vi "Multi-Instrument Controller.vi"() -> ()   [LabVIEW 2020]
uses:
  Typedefs/Instrument Control.ctl
  Typedefs/Save Params.ctl
  f5f9c0cd-fbfb-4a45-a1ff-eaef7659289b.vi
  <vilib>/Utility/xml.llb/Read From XML File(array).vi
  <vilib>/Utility/file.llb/Write Delimited Spreadsheet (string).vi
  <vilib>/Utility/xml.llb/Write to XML File(string).vi
  <vilib>/Comparison/Less/Less Functor/Less Functor.lvclass
  <instrlib>/Keithley 24XX/Keithley 24XX.lvlib
  <instrlib>/Keithley 648X Series/Keithley 648X Series.lvlib
  <instrlib>/Agilent 34405/Agilent 34405.lvlib
panel:
  out "XY Graph":cluster{dbl[], "Current":dbl[]}[](graph)
  out "rendezvous":T1
  out "Path":path
  in  "Trigger Hardware Address":refnum<visa-resource-name>
  in  "Trigger type":enum16{"Software", "Hardware"}(ring)
  out "start time":dbl
  out "DAQ Timer":string
  in  "Integration Speed":u16(ring)=100 items=["Fast (167µs, 3 digits)"=1, "Med (1.67ms, 4 digits)"=10, "Normal (16.74ms, 5 digits)"=100, "High Accuracy (167ms, 6 digits)"=1000]
  in  "Instrument Config":T2[](array[typedef])
  in  "Running":bool
  in  "Start":bool
  in  "Exit":bool
  in  "Number of Instruments":u64=1 min=1 max=32
  in  "Looping Mode":enum16{"Remote looping", "Local looping"}(ring)
  out "Filename":string
  in  "Stop":bool
  out "Iteration":i32
  in  "Number of Trials\nMax 2500 for remote":i16=300
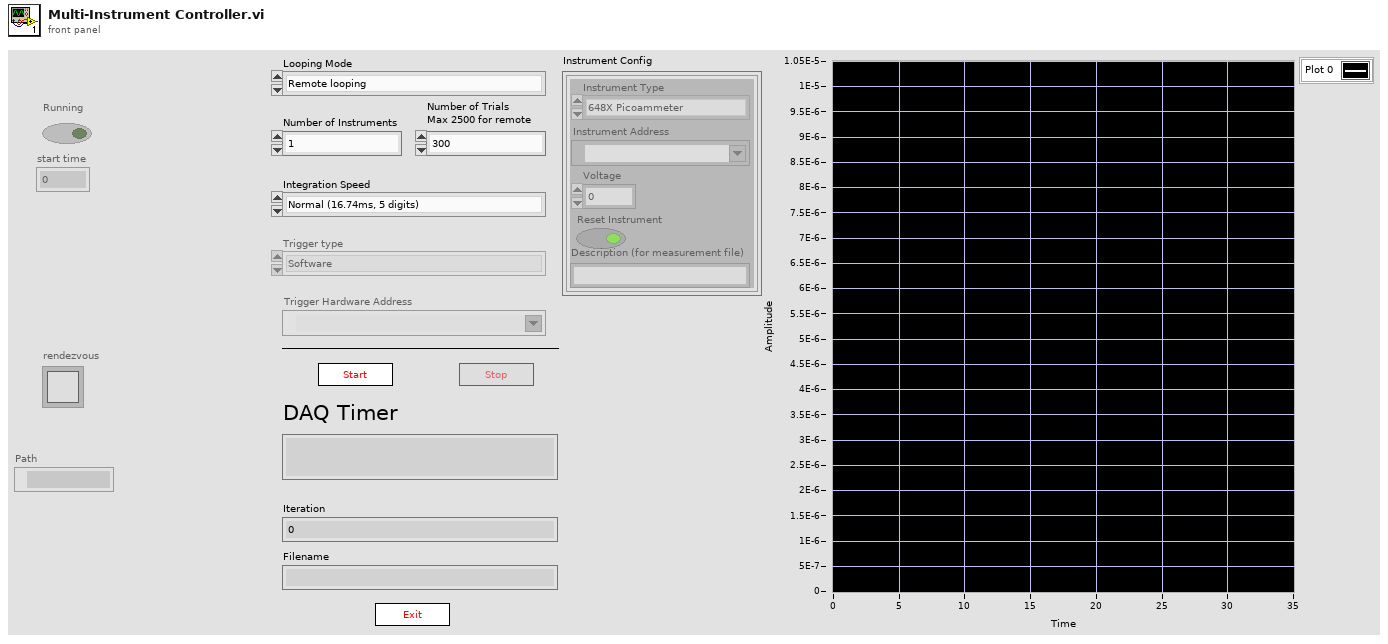
[diagram p1: front panel]
types:
  T1 = typedef "Rendezvous RefNum" = refnum<k1>
  T2 = typedef "Instrument Control.ctl" = cluster{"Instrument Address":refnum<visa-resource-name>, "Voltage":dbl, "Reset Instrument":bool, "Instrument Type":enum16{"648X Picoammeter", "24XX SMU", "237 SMU", "344XX DMM"}, "Description (for measurement file)":string}
  T3 = typedef "Save Params.ctl" = cluster{"Number of Instruments":u64, "Instrument Config":T2[], "Integration Speed":u16, "Measurement Mode":u16, "Number of Trials\nMax 2500 for remote":i16, "Trigger type":enum16{"Software", "Hardware"}, "Trigger Hardware Address":refnum<visa-resource-name>}
  T4 = enum8{"Enabled", "Disabled", "Disabled and Grayed Out"}
  T5 = typedef "LVDateTimeRec.ctl" = cluster{"fractional second":dbl, "second":i32, "minute":i32, "hour":i32, "day of month":i32, "month":i32, "year":i32, "day of week":i32, "day of year":i32, "DST":i32}
  T6 = enum16{"648X Picoammeter", "24XX SMU", "237 SMU", "344XX DMM"}
  T7 = cluster{i32, string[][], cluster{dbl[], "Voltage":sgl[]}, cluster{dbl[], "Current":dbl[]}}
  T8 = cluster{i32, string[][], cluster{dbl[], "Voltage":sgl[]}, cluster{dbl[], "Current":dbl[]}}[]
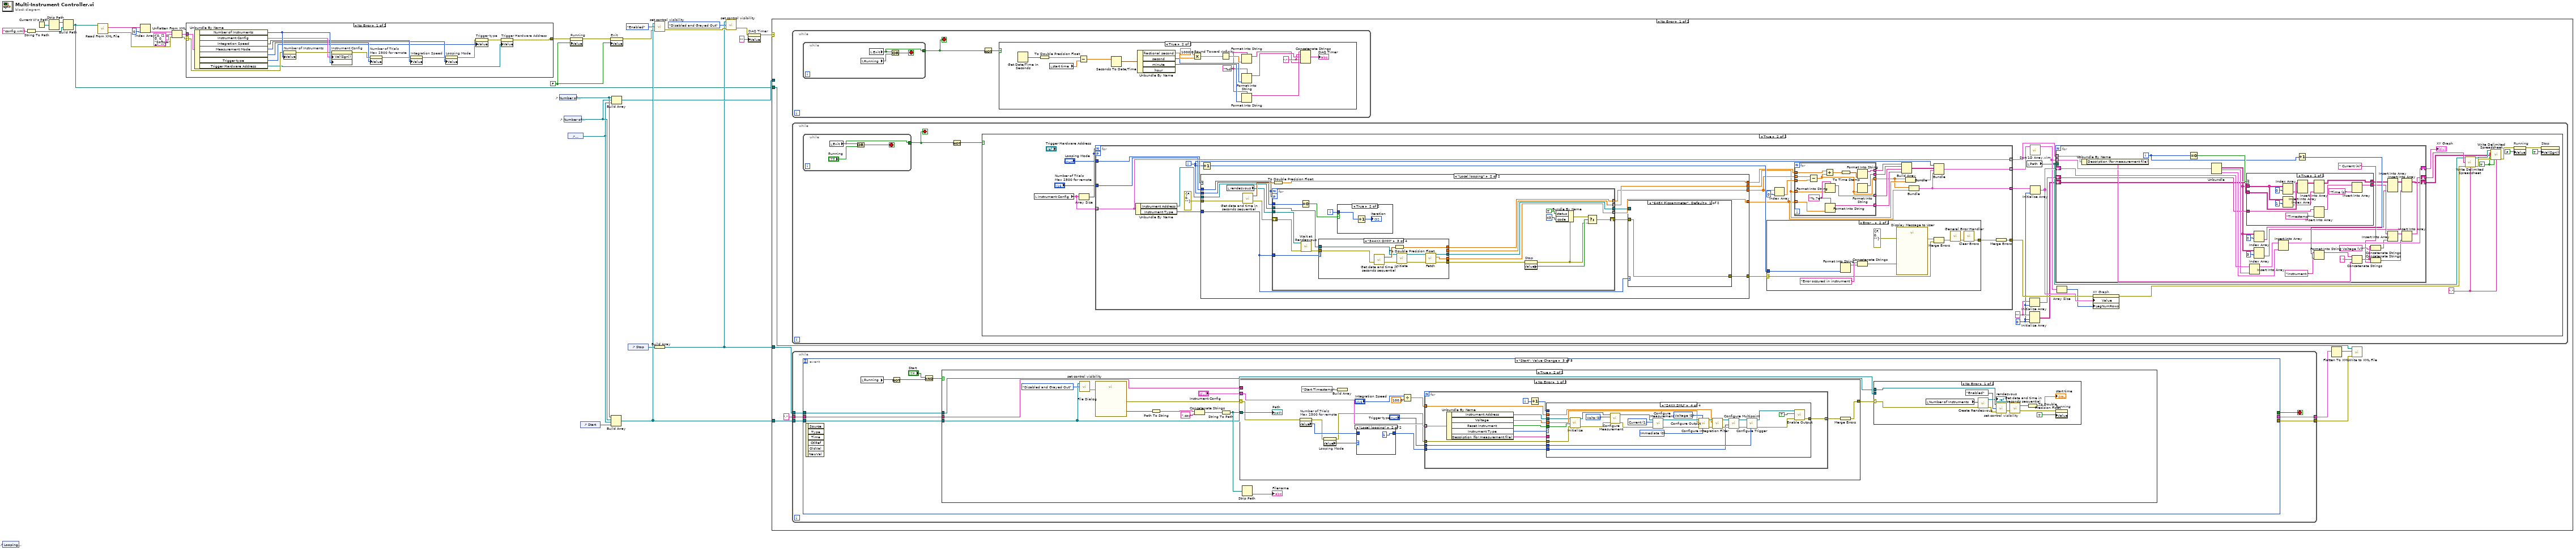
[diagram p0: block diagram]
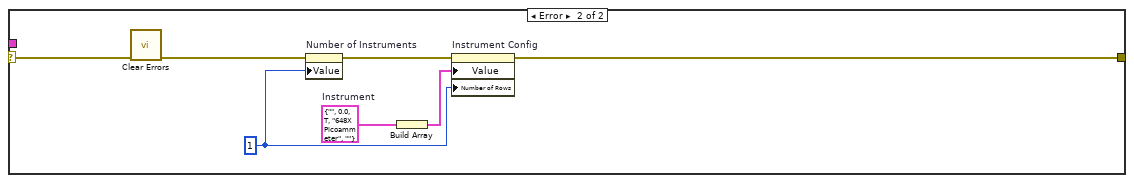
[diagram p2: hidden frame]
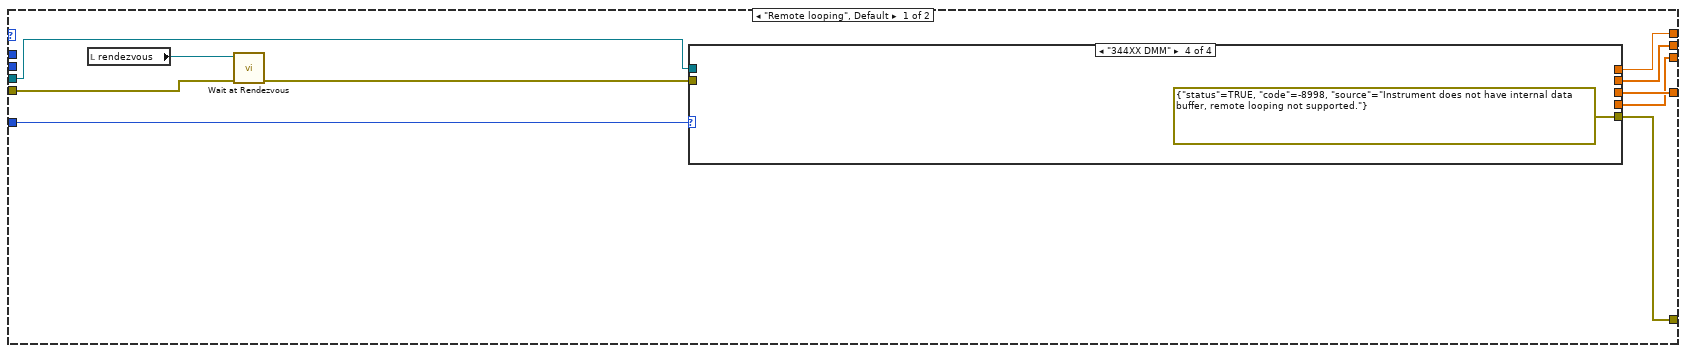
[diagram p6: hidden frame]
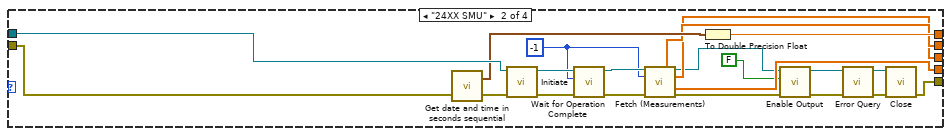
[diagram p8: hidden frame]
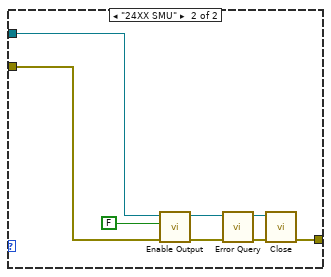
[diagram p10: hidden frame]
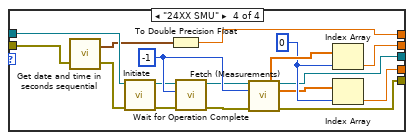
[diagram p13: hidden frame]
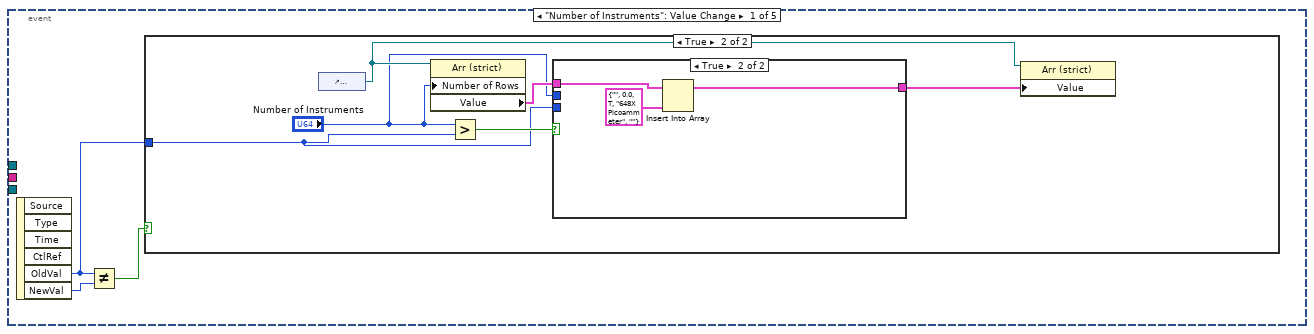
[diagram p16: hidden frame]
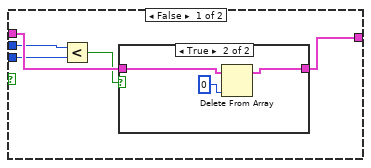
[diagram p18: hidden frame]
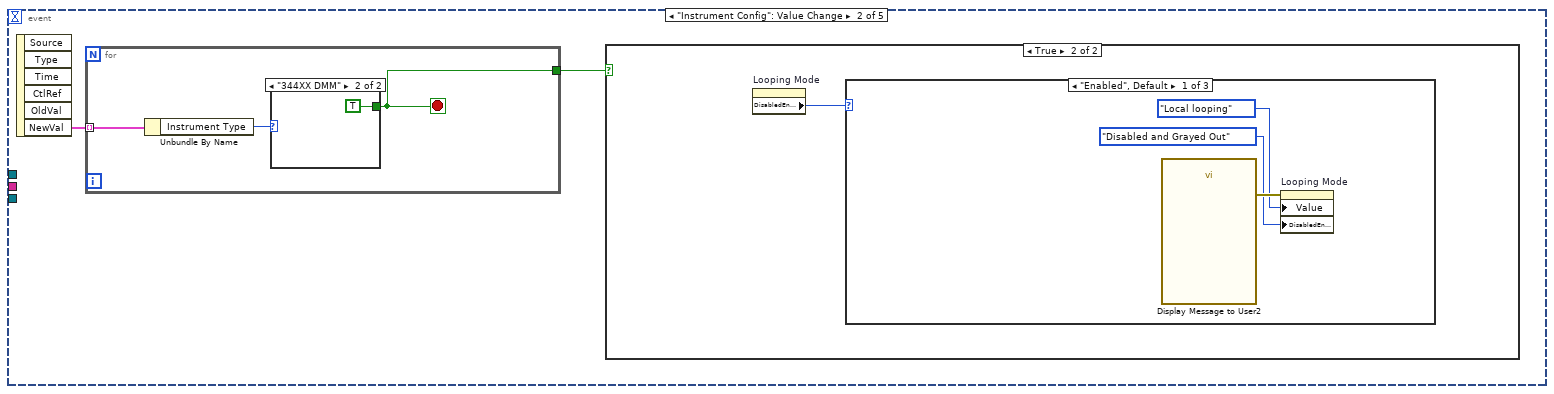
[diagram p20: hidden frame]
diagram:
  w15 = FALSE
  n1 = control-ref of="Looping Mode"() -> ()  [unwired: 1 out]
  n2 = String To Path(string="config.xml") -> (path=w13:path)
  n3 = Current VI's Path() -> (path=w20:path)
  n4 = Strip Path(path=w20) -> (stripped path=w19:path)  [unwired: 1 out]
  n5 = Build Path(base path=w19, name or relative path=w13) -> (appended path=w12:path)
  n6 = call-poly <vilib>:"Read From XML File.vi"("XML File Path"=w12) -> ("error out"=w2:errorcluster, "XML Elements"=w7:string[])  [unwired: 8 in, 1 out]
  n7 = Index Array(array=w7, index=0) -> (element=w4:string)
  n8 = Unflatten From XML(xml string=w4, type=T3 {"Number of Instruments"=0, "Instrument Config"=[], "Integration Speed"=0, "Measurement Mode"=0, "Number of Trials\nMax 2500 for remote"=0, "Trigger type"=enum."Software", "Trigger Hardware Address"=""} ("output cluster"), error in (no error)=w2) -> (value=w3:T3, error out=w1:errorcluster)
  n9 = case shown="No Error" w1 {
    selector: w1 -> [w37 w53]
    tunnel: [w32 w47] -> w9
    tunnel: w3 -> [w31 _]
    frame No Error {
      n10 = Unbundle By Name(w31) -> ("Number of Instruments"=w46:u64, "Instrument Config"=w44:T2[], "Integration Speed"=w40:u16, "Measurement Mode"=w38:u16, "Number of Trials\nMax 2500 for remote"=w42:i16, "Trigger type"=w36:enum16{"Software", "Hardware"}, "Trigger Hardware Address"=w35:refnum<visa-resource-name>)
      n11 = property on="Number of Instruments" class="DigNum (strict)"(error in=w37, "Value"=w46) -> (error out=w45:errorcluster)  [unwired: 1 in, 1 out]
      n12 = property on="Instrument Config" class="Arr (strict)"(error in=w45, "Val(Sgnl)"=w44, "Number of Rows"=w46) -> (error out=w43:errorcluster)  [unwired: 1 in, 1 out]
      n13 = property on="Number of Trials\nMax 2500 for remote" class="DigNum (strict)"(error in=w43, "Value"=w42) -> (error out=w41:errorcluster)  [unwired: 1 in, 1 out]
      n14 = property on="Integration Speed" class="Ring (strict)"(error in=w41, "Value"=w40) -> (error out=w39:errorcluster)  [unwired: 1 in, 1 out]
      n15 = property on="Looping Mode" class="Enum (strict)"(error in=w39, "Value"=w38) -> (error out=w34:errorcluster)  [unwired: 1 in, 1 out]
      n16 = property on="Trigger type" class="Enum (strict)"(error in=w34, "Value"=w36) -> (error out=w33:errorcluster)  [unwired: 1 in, 1 out]
      n17 = property on="Trigger Hardware Address" class="VISAName"(error in=w33, "Value"=w35) -> (error out=w32:errorcluster)  [unwired: 1 in, 1 out]
    }
    frame Error {
      w50 = T2 {"Instrument Address"="", "Voltage"=0.0, "Reset Instrument"=TRUE, "Instrument Type"=enum."648X Picoammeter", "Description (for measurement file)"=""}  # Instrument
      w51 = 1
      n18 = call <vilib>:"Clear Errors.vi"("error in (no error)"=w53) -> ("error out"=w52:errorcluster)  [unwired: 5 in, 1 out]
      n19 = property on="Number of Instruments" class="DigNum (strict)"(error in=w52, "Value"=w51) -> (error out=w48:errorcluster)  [unwired: 1 in, 1 out]
      n20 = Build Array(w50) -> (w49:T2[])
      n21 = property on="Instrument Config" class="Arr (strict)"(error in=w48, "Value"=w49, "Number of Rows"=w51) -> (error out=w47:errorcluster)  [unwired: 1 in, 1 out]
    }
  }
  n22 = control-ref of="Number of Instruments"() -> (w23:refnum<vi>)
  n23 = control-ref of="Number of Trials\nMax 2500 for remote"() -> (w22:refnum<vi>)
  n24 = control-ref of="Instrument Config"() -> (w21:refnum<vi>)
  n25 = property on="Running" class="Bool (strict)"(error in=w9, "Value"=w15) -> (error out=w14:errorcluster)  [unwired: 1 in, 1 out]
  n26 = control-ref of="Start"() -> (w29:refnum<vi>)
  n27 = property on="Exit" class="Bool (strict)"(error in=w14, "Value"=w15) -> (error out=w24:errorcluster)  [unwired: 1 in, 1 out]
  n28 = Build Array(w23, w22, w21, w29) -> (w25:refnum<vi>[])
  n29 = Build Array(w23, w22, w21) -> (w17:refnum<vi>[])
  n30 = control-ref of="Stop"() -> (w28:refnum<vi>)
  n31 = call "set control visibility.vi"("error in"=w24, "Disabled"=T4."Enabled", "Controls Reference Array"=w25) -> ("error out"=w27:errorcluster)  [unwired: 1 in]
  n32 = Build Array(w28) -> (w16:refnum<vi>[])
  n33 = call "set control visibility.vi"("error in"=w27, "Disabled"=T4."Disabled and Grayed Out", "Controls Reference Array"=w16) -> ("error out"=w8:errorcluster)  [unwired: 1 in]
  n34 = property on="DAQ Timer" class="Str"(error in=w8, "Value"="") -> (error out=w10:errorcluster)  [unwired: 1 in, 1 out]
  n35 = case shown="No Error" w10 {
    selector: w10 -> [_ w514]
    tunnel: w25 -> [w59 _]
    tunnel: w12 -> [w55 _]
    tunnel: w17 -> [_ _]
    tunnel: w16 -> [w54 _]
    frame No Error {
      n36 = while {
        stop <- w61 stop-if-true
        n37 = while {
          tunnel: [w80] -> w61
          stop <- w81 stop-if-true
          n38 = local read "Running"() -> (w82:bool)
          n39 = local read "Exit"() -> (w80:bool)
          n40 = Or(x=w80, y=w82) -> (x .or. y?=w81:bool)
        }
        n41 = Not(x=w61) -> (.not. x?=w62:bool)
        n42 = case shown="True" w62 {
          frame False {
          }
          frame True {
            w64 = "%d" ("format string")
            w69 = ":"
            n43 = Get Date/Time In Seconds() -> (seconds since 1Jan1904=w66:timestamp)
            n44 = To Double Precision Float(number=w66) -> (double precision float=w65:dbl)
            n45 = local read "start time"() -> (w63:dbl)
            n46 = Subtract(x=w65, y=w63) -> (x-y=w79:dbl)
            n47 = Seconds To Date/Time(time stamp (now)=w79) -> (date time rec=w78:T5)  [unwired: 1 in]
            n48 = Unbundle By Name(w78) -> ("fractional second"=w77:dbl, "second"=w73:i32, "minute"=w72:i32)  [unwired: 1 out]
            n49 = Multiply(x=1000.0, y=w77) -> (x*y=w75:dbl)
            n50 = Round Toward -Infinity(1:w75) -> (0:w74:dbl)
            n51 = Format Into String(format string=w64, w74) -> (resulting string=w68:string)  [unwired: 2 in, 1 out]
            n52 = Format Into String(format string=w64, w73) -> (resulting string=w70:string)  [unwired: 2 in, 1 out]
            n53 = Format Into String(format string=w64, w72) -> (resulting string=w71:string)  [unwired: 2 in, 1 out]
            n54 = Concatenate Strings(w71, w69, w70, w69, w68) -> (→"DAQ Timer":string)
          }
        }
      }
      n55 = while {
        stop <- w83 stop-if-true
        n56 = while {
          tunnel: [w316] -> w83
          stop <- w317 stop-if-true
          n57 = local read "Exit"() -> (w316:bool)
          n58 = Or(x=w316, y="Running") -> (x .or. y?=w317:bool)
        }
        n59 = Not(x=w83) -> (.not. x?=w84:bool)
        n60 = case shown="True" w84 {
          frame False {
          }
          frame True {
            w90 = ","
            w92 = TRUE ("transpose? (no:F)")
            w87 = ""
            w86 = 0 ("dimension size")
            n61 = local read "Instrument Config"() -> (w111:T2[])
            n62 = Array Size(array=w111) -> (size(s)=w112:i32)
            n63 = for {
              N: w112 -> [_]
              workers-P: w112 -> [_]
              tunnel: w111 -> [w172] mode=indexing
              tunnel: [w175] -> w100
              tunnel: [w173] -> w110 mode=indexing
              tunnel: [w172] -> w109 mode=indexing
              tunnel: "Looping Mode" -> [w171]
              tunnel: "Number of Trials\nMax 2500 for remote" -> [w170]
              tunnel: [w164] -> w103
              i -> [w169]
              n64 = Unbundle By Name(w172) -> ("Instrument Address"=w163:refnum<visa-resource-name>, "Instrument Type"=w161:T6)
              n65 = case shown="\"Local looping\"" w171 {
                tunnel: w163 -> [w191 w227]
                tunnel: [w190 w231] -> w184
                tunnel: [w189 w230] -> w168
                tunnel: [w188 w229] -> w166
                tunnel: [w187 w228] -> w182
                tunnel: errorcluster {"status"=FALSE, "code"=0, "source"=""} ("error constant") -> [w195 w226]
                tunnel: [w186 w221] -> w160
                tunnel: w170 -> [_ w219]
                tunnel: w169 -> [_ w223]
                tunnel: w161 -> [w193 w220]
                frame "Remote looping", Default {
                  n66 = local read "rendezvous"() -> (w194:T1)
                  n67 = call <vilib>:"Wait at Rendezvous.vi"("error in (no error)"=w195, "rendezvous"=w194) -> ("error out"=w192:errorcluster)  [unwired: 3 in, 2 out]
                  n68 = case shown="\"344XX DMM\"" w193 {
                    tunnel: w192 -> [_ w198 _ _]
                    tunnel: w191 -> [_ w216 _ _]
                    tunnel: [_ w214 _ _] -> w190
                    tunnel: [_ w210 _ _] -> w189
                    tunnel: [_ w209 _ _] -> w188
                    tunnel: [_ w208 _ _] -> w187
                    tunnel: [_ w199 _ errorcluster {"status"=TRUE, "code"=-8998, "source"="Instrument does not have internal data buffer, remote looping not supported."} ("error constant")] -> w186
                    frame "648X Picoammeter", Default {
                    }
                    frame "24XX SMU" {
                      w207 = -1
                      n69 = call "Get date and time in seconds sequential.vi"("error in (no error)"=w198) -> ("error out"=w197:errorcluster, "current time"=w215:timestamp)  [unwired: 1 in]
                      n70 = call <instrlib>:"Initiate.vi"("error in (no error)"=w197, "VISA resource name"=w216) -> ("error out"=w196:errorcluster, "VISA resource name out"=w213:refnum<visa-resource-name>)  [unwired: 8 in]
                      n71 = call <instrlib>:"Wait for Operation Complete.vi"("error in (no error)"=w196, "Timeout (10000 ms)"=w207, "VISA resource name"=w213) -> ("error out"=w211:errorcluster, "VISA resource name out"=w212:refnum<visa-resource-name>)  [unwired: 7 in]
                      n72 = call <instrlib>:"Fetch (Measurements).vi"("VISA resource name"=w212, "Timeout (10000 ms)"=w207, "error in (no error)"=w211) -> ("Voltage"=w210:sgl[], "VISA resource name out"=w206:refnum<visa-resource-name>, "Current"=w209:sgl[], "Timestamp"=w208:sgl[], "error out"=w205:errorcluster)  [unwired: 6 in, 2 out]
                      n73 = To Double Precision Float(number=w215) -> (double precision float=w214:dbl)
                      n74 = call <instrlib>:"Enable Output.vi"("error in (no error)"=w205, "Enable Output (T: Enable)"=FALSE, "VISA resource name"=w206) -> ("error out"=w202:errorcluster, "VISA resource name out"=w203:refnum<visa-resource-name>)  [unwired: 7 in]
                      n75 = call <instrlib>:"Error Query.vi"("error in (no error)"=w202, "VISA resource name"=w203) -> ("error out"=w200:errorcluster, "VISA resource name out"=w201:refnum<visa-resource-name>)  [unwired: 6 in, 2 out]
                      n76 = call <instrlib>:"Close.vi"("error in (no error)"=w200, "VISA resource name"=w201) -> ("error out"=w199:errorcluster)  [unwired: 9 in]
                    }
                    frame "237 SMU" {
                    }
                    frame "344XX DMM" {
                    }
                  }
                }
                frame "Local looping" {
                  n77 = local read "rendezvous"() -> (w224:T1)
                  n78 = call "Get date and time in seconds sequential.vi"("error in (no error)"=w226) -> ("error out"=w225:errorcluster, "current time"=w232:timestamp)  [unwired: 1 in]
                  n79 = for {
                    N: w219 -> [_]
                    tunnel: [w260] -> w230 mode=indexing
                    tunnel: [w259] -> w229 mode=indexing
                    tunnel: [w252] -> w228 mode=indexing
                    tunnel: w227 -> [w258]
                    tunnel: [w257] -> w222
                    tunnel: w224 -> [w251]
                    tunnel: w223 -> [w255]
                    tunnel: w220 -> [w253]
                    workers-P: w219 -> [_]
                    shift-right: [w244] -> w218
                    shift-left: w225 -> [w250]
                    i -> [w256]
                    n80 = Equal To 0?(x=w255) -> (x = 0?=w254:bool)
                    n81 = call <vilib>:"Wait at Rendezvous.vi"("error in (no error)"=w250, "rendezvous"=w251) -> ("error out"=w249:errorcluster)  [unwired: 3 in, 2 out]
                    n82 = case shown="\"344XX DMM\"" w253 {
                      tunnel: w249 -> [w261 w262 w265 w275]
                      tunnel: [_ _ _ w286] -> w260
                      tunnel: [_ _ w267 w283] -> w259
                      tunnel: w258 -> [_ _ w269 w282]
                      tunnel: [_ _ w268 w279] -> w257
                      tunnel: [w261 w262 w266 w278] -> w248
                      tunnel: [_ _ w271 w276] -> w252
                      frame "648X Picoammeter", Default {
                      }
                      frame "237 SMU" {
                      }
                      frame "344XX DMM" {
                        n83 = call "Get date and time in seconds sequential.vi"("error in (no error)"=w265) -> ("error out"=w264:errorcluster, "current time"=w272:timestamp)  [unwired: 1 in]
                        n84 = To Double Precision Float(number=w272) -> (double precision float=w271:dbl)
                        n85 = call <instrlib>:"Initiate.vi"("error in (no error)"=w264, "VISA resource name"=w269) -> ("error out"=w263:errorcluster, "VISA resource name out"=w270:refnum<visa-resource-name>)  [unwired: 8 out]
                        n86 = call <instrlib>:"Fetch.vi"("error in (no error)"=w263, "VISA resource name"=w270) -> ("error out"=w266:errorcluster, "Measurement"=w267:dbl, "VISA resource name out"=w268:refnum<visa-resource-name>)  [unwired: 7 out]
                      }
                      frame "24XX SMU" {
                        w285 = 0
                        w288 = -1
                        n87 = call "Get date and time in seconds sequential.vi"("error in (no error)"=w275) -> ("error out"=w274:errorcluster, "current time"=w277:timestamp)  [unwired: 1 in]
                        n88 = call <instrlib>:"Initiate.vi"("error in (no error)"=w274, "VISA resource name"=w282) -> ("error out"=w273:errorcluster, "VISA resource name out"=w281:refnum<visa-resource-name>)  [unwired: 8 in]
                        n89 = To Double Precision Float(number=w277) -> (double precision float=w276:dbl)
                        n90 = call <instrlib>:"Wait for Operation Complete.vi"("error in (no error)"=w273, "Timeout (10000 ms)"=w288, "VISA resource name"=w281) -> ("error out"=w289:errorcluster, "VISA resource name out"=w280:refnum<visa-resource-name>)  [unwired: 7 in]
                        n91 = call <instrlib>:"Fetch (Measurements).vi"("VISA resource name"=w280, "Timeout (10000 ms)"=w288, "error in (no error)"=w289) -> ("Voltage"=w287:sgl[], "VISA resource name out"=w279:refnum<visa-resource-name>, "Current"=w284:sgl[], "error out"=w278:errorcluster)  [unwired: 6 in, 3 out]
                        n92 = Index Array(array=w287, index=w285) -> (element=w286:sgl)
                        n93 = Index Array(array=w284, index=w285) -> (element=w283:sgl)
                      }
                    }
                    n94 = case shown="True" w254 {
                      tunnel: w256 -> [_ w291]
                      frame False {
                      }
                      frame True {
                        n95 = Increment(x=w291) -> (x+1=→"Iteration":i32)
                      }
                    }
                    n96 = property on="Stop" class="Bool (strict)"(error in=w248) -> (error out=w243:errorcluster, "Value"=w247:bool)  [unwired: 1 in, 1 out]
                    n97 = Bundle By Name(cluster=w243, "status"=TRUE, "code"=43) -> (w242:errorcluster)
                    n98 = Select(t=w242, s=w247, f=w243) -> (s? t:f=w244:errorcluster)
                  }
                  n99 = To Double Precision Float(number=w232) -> (double precision float=w231:dbl)
                  n100 = case shown="\"648X Picoammeter\", Default" w220 {
                    tunnel: w222 -> [_ w237]
                    tunnel: [w233 w236] -> w221
                    tunnel: w218 -> [w233 w234]
                    frame "648X Picoammeter", Default {
                    }
                    frame "24XX SMU" {
                      n101 = call <instrlib>:"Enable Output.vi"("error in (no error)"=w234, "Enable Output (T: Enable)"=FALSE, "VISA resource name"=w237) -> ("error out"=w240:errorcluster, "VISA resource name out"=w241:refnum<visa-resource-name>)  [unwired: 7 in]
                      n102 = call <instrlib>:"Error Query.vi"("error in (no error)"=w240, "VISA resource name"=w241) -> ("error out"=w238:errorcluster, "VISA resource name out"=w239:refnum<visa-resource-name>)  [unwired: 6 in, 2 out]
                      n103 = call <instrlib>:"Close.vi"("error in (no error)"=w238, "VISA resource name"=w239) -> ("error out"=w236:errorcluster)  [unwired: 9 in]
                    }
                  }
                }
              }
              n104 = Increment(x=w169) -> (x+1=w185:i32)
              n105 = case shown="Error .." w160 {
                selector: w160 -> [w305 w309]
                tunnel: [w305 w306] -> w180
                tunnel: w185 -> [_ w314]
                frame No Error {
                }
                frame Error {
                  n106 = Format Into String(w314) -> (resulting string=w313:string)  [unwired: 3 in, 1 out]
                  n107 = Concatenate Strings("Error occured in instrument " ("Message"), w313) -> (w312:string)
                  n108 = call "Display Message to User"("error in (no error)"=errorcluster {"status"=FALSE, "code"=0, "source"=""} ("error constant"), "Message"=w312) -> ("error out"=w310:errorcluster)  [unwired: 8 in, 1 out]
                  n109 = Merge Errors(w310, w309) -> (w308:errorcluster)
                  n110 = call <vilib>:"General Error Handler.vi"("error in (no error)"=w308) -> ("error out"=w307:errorcluster)  [unwired: 10 in, 4 out]
                  n111 = call <vilib>:"Clear Errors.vi"("error in (no error)"=w307) -> ("error out"=w306:errorcluster)  [unwired: 5 in, 1 out]
                }
              }
              n112 = Index Array(array=w182, index=0) -> (element=w181:dbl)
              n113 = for {
                tunnel: [w304] -> w176 mode=indexing
                tunnel: [w303] -> w177 mode=indexing
                tunnel: w182 -> [w302] mode=indexing
                tunnel: w168 -> [w292] mode=indexing
                tunnel: w181 -> [w301]
                tunnel: w166 -> [w294] mode=indexing
                tunnel: w184 -> [w299]
                tunnel: [w296] -> w179 mode=indexing
                tunnel: [w295] -> w178 mode=indexing
                tunnel: [w293] -> w167 mode=indexing
                w300 = "%.7e"
                n114 = Subtract(x=w302, y=w301) -> (x-y=w293:dbl)
                n115 = Add(x=w299, y=w293) -> (x+y=w298:dbl)
                n116 = Format Into String(format string=w300, w292) -> (resulting string=w303:string)  [unwired: 2 in, 1 out]
                n117 = Format Into String(format string=w300, w294) -> (resulting string=w304:string)  [unwired: 2 in, 1 out]
                n118 = To Time Stamp(1:w298) -> (0:w297:timestamp)
                n119 = Format Into String(w297) -> (resulting string=w296:string)  [unwired: 3 in, 1 out]
                n120 = Format Into String(w293) -> (resulting string=w295:string)  [unwired: 3 in, 1 out]
              }
              n121 = Build Array(w179, w178, w177, w176) -> (w174:string[][])
              n122 = Bundle(w167, "Voltage"=w168) -> (w165:cluster{dbl[], "Voltage":sgl[]})  [unwired: 1 in]
              n123 = Bundle(w167, "Current"=w166) -> (w164:cluster{dbl[], "Current":dbl[]})  [unwired: 1 in]
              n124 = Bundle(w169, w174, w165, w164) -> (w173:T7)  [unwired: 1 in]
              n125 = Merge Errors(w180) -> (w175:errorcluster)
            }
            n126 = local read "Path"() -> (w94:path)
            n127 = Initialize Array(w87, w86) -> (w97:string[])
            n128 = Initialize Array(w87, w86, w86) -> (w88:string[][])
            n129 = call "Sort 1D Array.vim"("unsorted array"=w110) -> ("sorted array"=w99:T8)  [unwired: 10 in]
            n130 = Initialize Array(w103, w86) -> (w101:cluster{dbl[], "Current":dbl[]}[])
            n131 = for {
              tunnel: w99 -> [w144] mode=indexing
              tunnel: w109 -> [w143] mode=indexing
              tunnel: w94 -> [_]
              shift-right: [w133] -> w102
              shift-left: w101 -> [w137]
              shift-right: [w122] -> w95
              shift-left: w97 -> [w127]
              shift-right: [w113] -> w85
              shift-left: w88 -> [w121]
              i -> [w128]
              n132 = Unbundle By Name(w143) -> ("Description (for measurement file)"=w131:string)
              n133 = Equal To 0?(x=w128) -> (x = 0?=w129:bool)
              n134 = Unbundle(w144) -> (w117:string[][], w136:cluster{dbl[], "Voltage":sgl[]}, w134:cluster{dbl[], "Current":dbl[]})  [unwired: 1 out]
              n135 = case shown="True" w129 {
                tunnel: w127 -> [w146 w159]
                tunnel: [w146 w155] -> w126
                tunnel: w121 -> [w145 w154]
                tunnel: [w145 w152] -> w118
                tunnel: w117 -> [_ w147]
                frame False {
                }
                frame True {
                  n136 = Index Array(array=w147, index (row)=0) -> (element=w150:string[])  [unwired: 1 in]
                  n137 = Index Array(array=w147, index (row)=1) -> (element=w148:string[])  [unwired: 1 in]
                  n138 = Insert Into Array(array=w154, new element=w150) -> (w153:string[][])  [unwired: 2 in]
                  n139 = Insert Into Array(array=w153, new element=w148) -> (w152:string[][])  [unwired: 2 in]
                  n140 = Insert Into Array(array=w159, new element="Timestamp") -> (w157:string[])  [unwired: 1 in]
                  n141 = Insert Into Array(array=w157, new element="Time (s)") -> (w155:string[])  [unwired: 1 in]
                }
              }
              n142 = Insert Into Array(array=w137, new element=w136) -> (w135:cluster{dbl[], "Current":dbl[]}[])  [unwired: 1 in]
              n143 = Index Array(array=w117, index (row)=2) -> (element=w116:string[])  [unwired: 1 in]
              n144 = Index Array(array=w117, index (row)=3) -> (element=w114:string[])  [unwired: 1 in]
              n145 = Insert Into Array(array=w135, new element=w134) -> (w133:cluster{dbl[], "Current":dbl[]}[])  [unwired: 1 in]
              n146 = Increment(x=w128) -> (x+1=w142:i32)
              n147 = Format Into String(initial string="Instrument ", w142) -> (resulting string=w140:string)  [unwired: 2 in, 1 out]
              n148 = Concatenate Strings(w140, " ", w131) -> (w138:string)
              n149 = Concatenate Strings(w138, " Voltage (V)") -> (w125:string)
              n150 = Concatenate Strings(w138, " Current (A)") -> (w124:string)
              n151 = Insert Into Array(array=w118, new element=w116) -> (w115:string[][])  [unwired: 2 in]
              n152 = Insert Into Array(array=w126, new element=w125) -> (w123:string[])  [unwired: 1 in]
              n153 = Insert Into Array(array=w115, new element=w114) -> (w113:string[][])  [unwired: 2 in]
              n154 = Insert Into Array(array=w123, new element=w124) -> (w122:string[])  [unwired: 1 in]
            }
            "XY Graph" <- w102
            n155 = Array Size(array=w99) -> (size(s)=w98:i32)
            n156 = property on="XY Graph" class="XYGraph (strict)"(error in=w100, "Value"=w101, "LegNumRows"=w98) -> (error out=w96:errorcluster)  [unwired: 1 in, 1 out]
            n157 = call-poly <vilib>:"Write Delimited Spreadsheet.vi"("file path (dialog if empty)"=w94, "1D data"=w95, "error in (no error)"=w96, "delimiter (\\t)"=w90) -> ("new file path (Not A Path if cancelled)"=w91:path, "error out"=w93:errorcluster)  [unwired: 10 in]
            n158 = call-poly <vilib>:"Write Delimited Spreadsheet.vi"("file path (dialog if empty)"=w91, "2D data"=w85, "append to file? (new file:F)"=w92, "error in (no error)"=w93, "transpose? (no:F)"=w92, "delimiter (\\t)"=w90) -> ("error out"=w89:errorcluster)  [unwired: 8 in, 1 out]
            n159 = property on="Running" class="Bool (strict)"(error in=w89, "Value"=FALSE) -> (error out=w106:errorcluster)  [unwired: 1 in, 1 out]
            n160 = property on="Stop" class="Bool (strict)"(error in=w106, "Val(Sgnl)"=TRUE) -> ()  [unwired: 1 in, 2 out]
          }
        }
      }
      n161 = while {
        tunnel: "," -> [w323]
        tunnel: w59 -> [w322]
        tunnel: [w321] -> w58
        tunnel: [w320] -> w56
        tunnel: w54 -> [w319]
        stop <- w324 stop-if-true
        n162 = event shown="[2] \"Start\": Value Change" {
          selector: _ -> [_ _ _ _ _]
          dyn-events: _ -> [_ _ _ _ _]
          timeout: _ -> [_ _ _ _ _]
          tunnel: [_ _ _ _ "Exit"] -> w324
          tunnel: w323 -> [_ _ w360 _ _]
          tunnel: w322 -> [_ _ w359 w471 _]
          tunnel: [_ _ _ _ w507] -> w321
          tunnel: [_ _ _ _ errorcluster {"status"=FALSE, "code"=0, "source"=""} ("error constant")] -> w320
          tunnel: w319 -> [_ _ w358 w467 _]
          event "Number of Instruments": Value Change {
            n163 = event-data() -> ("OldVal"=w325:u64, "NewVal"=w327:u64)  [unwired: 1 in, 4 out]
            n164 = Not Equal?(x=w325, y=w327) -> (x != y?=w326:bool)
            n165 = case shown="True" w326 {
              tunnel: w325 -> [_ w328]
              frame False {
              }
              frame True {
                n166 = control-ref of="Instrument Config"() -> (w330:refnum<vi>)
                n167 = property on="Property Node" class="Arr (strict)"(reference=w330, "Number of Rows"="Number of Instruments") -> ("Value"=w332:T2[])  [unwired: 1 in, 2 out]
                n168 = Greater?(x="Number of Instruments", y=w328) -> (0:w333:bool)
                n169 = case shown="True" w333 {
                  tunnel: w332 -> [w338 w345]
                  tunnel: [w337 w344] -> w331
                  tunnel: "Number of Instruments" -> [w336 _]
                  tunnel: w328 -> [w335 _]
                  frame False {
                    n170 = Less?(x=w336, y=w335) -> (x < y?=w334:bool)
                    n171 = case shown="True" w334 {
                      tunnel: w338 -> [w339 w342]
                      tunnel: [w339 w341] -> w337
                      frame False {
                      }
                      frame True {
                        n172 = Delete From Array(array=w342, index=0) -> (array with subset deleted=w341:T2[])  [unwired: 1 in, 1 out]
                      }
                    }
                  }
                  frame True {
                    n173 = Insert Into Array(array=w345, new element=T2 {"Instrument Address"="", "Voltage"=0.0, "Reset Instrument"=TRUE, "Instrument Type"=enum."648X Picoammeter", "Description (for measurement file)"=""}) -> (w344:T2[])  [unwired: 1 in]
                  }
                }
                n174 = property on="Property Node" class="Arr (strict)"(reference=w330, "Value"=w331) -> ()  [unwired: 1 in, 2 out]
              }
            }
          }
          event "Instrument Config": Value Change {
            n175 = event-data() -> ("NewVal"=w347:T2[])  [unwired: 1 in, 5 out]
            n176 = for {
              tunnel: w347 -> [w355] mode=indexing
              tunnel: [w353] -> w346
              stop <- w353 stop-if-true
              n177 = Unbundle By Name(w355) -> ("Instrument Type"=w354:T6)
              n178 = case shown="\"344XX DMM\"" w354 {
                tunnel: [FALSE TRUE] -> w353
                frame "648X Picoammeter", Default {
                }
                frame "344XX DMM" {
                }
              }
            }
            n179 = case shown="True" w346 {
              frame False {
                n180 = property on="Looping Mode" class="Enum (strict)"("DisabledEnum"=T4."Enabled" ("Disabled")) -> ()  [unwired: 2 in, 2 out]
              }
              frame True {
                n181 = property on="Looping Mode" class="Enum (strict)"() -> ("DisabledEnum"=w349:T4)  [unwired: 2 in, 2 out]
                n182 = case shown="\"Enabled\", Default" w349 {
                  frame "Enabled", Default {
                    n183 = call "Display Message to User2"() -> ("error out"=w352:errorcluster)  [unwired: 10 in, 1 out]
                    n184 = property on="Looping Mode" class="Enum (strict)"(error in=w352, "Value"=enum16{"Remote looping", "Local looping"}."Local looping" ("Looping Mode"), "DisabledEnum"=T4."Disabled and Grayed Out" ("Disabled")) -> ()  [unwired: 1 in, 2 out]
                  }
                  frame "Disabled" {
                  }
                  frame "Disabled and Grayed Out" {
                  }
                }
              }
            }
          }
          event "Start": Value Change {
            n185 = event-data() -> ()  [unwired: 1 in, 6 out]
            n186 = local read "Running"() -> (w364:bool)
            n187 = Not(x=w364) -> (.not. x?=w363:bool)
            n188 = And(x="Start", y=w363) -> (x .and. y?=w361:bool)
            n189 = case shown="True" w361 {
              tunnel: w360 -> [_ w372]
              tunnel: w359 -> [_ w367]
              tunnel: w358 -> [_ w366]
              frame False {
              }
              frame True {
                n190 = call "set control visibility.vi"("Disabled"=T4."Disabled and Grayed Out", "Controls Reference Array"=w367) -> ("error out"=w369:errorcluster)  [unwired: 2 in]
                n191 = call "File Dialog"("error in"=w369) -> ("selected path"=w375:path, "error out"=w373:errorcluster)  [unwired: 11 in, 2 out]
                n192 = Path To String(path=w375) -> (string=w378:string)
                n193 = Concatenate Strings(w378, ".csv") -> (w376:string)
                n194 = String To Path(string=w376) -> (path=w371:path)
                n195 = case shown="No Error" w373 {
                  selector: w373 -> [w400 w466]
                  tunnel: "Instrument Config" -> [w409 _]
                  tunnel: w372 -> [_ _]
                  tunnel: w371 -> [w403 _]
                  tunnel: [w401 w466] -> w365
                  frame No Error {
                    n196 = property on="Number of Trials\nMax 2500 for remote" class="DigNum (strict)"(error in=w400) -> (error out=w396:errorcluster, "Value"=w399:i16)  [unwired: 1 in, 1 out]
                    n197 = property on="Looping Mode" class="Enum (strict)"(error in=w396) -> (error out=w395:errorcluster, "Value"=w397:enum16{"Remote looping", "Local looping"})  [unwired: 1 in, 1 out]
                    n198 = Build Array("Start Timestamp") -> ()  [unwired: 1 out]
                    n199 = case shown="\"Local looping\"" w397 {
                      tunnel: [w410 1] -> w398
                      tunnel: w399 -> [w410 _]
                      frame "Remote looping", Default {
                      }
                      frame "Local looping" {
                      }
                    }
                    n200 = Divide(x="Integration Speed", y=100.0) -> (x/y=w404:dbl)
                    n201 = for {
                      tunnel: w409 -> [w424] mode=indexing
                      tunnel: [w420] -> w408 mode=indexing
                      tunnel: w395 -> [w422]
                      tunnel: w404 -> [w414]
                      tunnel: "Trigger type" -> [w413]
                      tunnel: w398 -> [w412]
                      i -> [w418]
                      n202 = Unbundle By Name(w424) -> ("Instrument Address"=w416:refnum<visa-resource-name>, "Voltage"=w421:dbl, "Reset Instrument"=w423:bool, "Instrument Type"=w419:T6, "Description (for measurement file)"=w415:string)
                      n203 = Increment(x=w418) -> (x+1=w417:i32)
                      n204 = case shown="\"24XX SMU\"" w419 {
                        tunnel: w423 -> [w427 _ w437 w459]
                        tunnel: w422 -> [_ _ w436 w454]
                        tunnel: w421 -> [_ _ _ w453]
                        tunnel: [w426 errorcluster {"status"=TRUE, "code"=-8999, "source"="Instrument not yet implemented"} ("error constant") w430 w442] -> w420
                        tunnel: w417 -> [_ _ _ _]
                        tunnel: w416 -> [w428 _ w438 w449]
                        tunnel: w415 -> [_ _ _ _]
                        tunnel: w414 -> [_ _ _ w451]
                        tunnel: w413 -> [_ _ _ w440]
                        tunnel: w412 -> [_ _ _ w439]
                        frame "648X Picoammeter", Default {
                          n205 = call <instrlib>:"Initialize.vi"("error in (no error)"=errorcluster {"status"=TRUE, "code"=-8999, "source"="Instrument not yet implemented"} ("error constant"), "Reset (True)"=w427, "VISA resource name"=w428) -> ("error out"=w426:errorcluster)  [unwired: 7 in, 1 out]
                        }
                        frame "237 SMU" {
                        }
                        frame "344XX DMM" {
                          w433 = 2 items=["DC Volts", "AC Volts", "DC Current", "AC Current", "2-Wire Resistance", "Frequency", "Temperature", "Capacitance", "Continuity", "Diode", "4-Wire Resistance", "2nd DC Volts", "2nd AC Volts", "2nd DC Current", "2nd AC Current", "2nd Frequency"] ("Function (0: DC Volts)")
                          n206 = call <instrlib>:"Initialize.vi"("error in (no error)"=w436, "Reset (True)"=w437, "VISA resource name"=w438) -> ("error out"=w434:errorcluster, "VISA resource name out"=w435:refnum<visa-resource-name>)  [unwired: 6 in, 1 out]
                          n207 = call <instrlib>:"Configure Measurement.vi"("error in (no error)"=w434, "Function (0: DC Volts)"=w433, "VISA resource name"=w435) -> ("error out"=w431:errorcluster, "VISA resource name out"=w432:refnum<visa-resource-name>)  [unwired: 7 in]
                          n208 = call <instrlib>:"Configure Trigger.vi"("error in (no error)"=w431, "VISA resource name"=w432) -> ("error out"=w430:errorcluster)  [unwired: 1 in, 8 out]
                        }
                        frame "24XX SMU" {
                          w457 = u16 0 items=["Immediate", "Triggered"] ("Output Type  (0: Immediate)")
                          w458 = u16 0 items=["Voltage", "Current"] ("Source Mode  (0: Voltage)")
                          w462 = u16 0 items=["Volts", "Current", "Resistance"] ("Function (0: Volts)")
                          w465 = u16 1 items=["Volts", "Current", "Resistance"] ("Function (0: Volts)")
                          n209 = call <instrlib>:"Initialize.vi"("error in (no error)"=w454, "Reset (True)"=w459, "VISA resource name"=w449) -> ("error out"=w463:errorcluster, "VISA resource name out"=w464:refnum<visa-resource-name>)  [unwired: 5 in, 2 out]
                          n210 = call <instrlib>:"Configure Measurement.vi"("error in (no error)"=w463, "Function (0: Volts)"=w462, "VISA resource name"=w464) -> ("error out"=w460:errorcluster, "VISA resource name out"=w461:refnum<visa-resource-name>)  [unwired: 7 in]
                          n211 = call <instrlib>:"Configure Measurement.vi"("error in (no error)"=w460, "Function (0: Volts)"=w465, "VISA resource name"=w461) -> ("error out"=w456:errorcluster, "VISA resource name out"=w455:refnum<visa-resource-name>)  [unwired: 7 in]
                          n212 = call <instrlib>:"Configure Output.vi"("Output Type  (0: Immediate)"=w457, "Source Mode  (0: Voltage)"=w458, "error in (no error)"=w456, "Output Level (0)"=w453, "VISA resource name"=w455) -> ("error out"=w450:errorcluster, "VISA resource name out"=w452:refnum<visa-resource-name>)  [unwired: 5 in]
                          n213 = call <instrlib>:"Configure Integration Filter.vi"("error in (no error)"=w450, "Measurement Speed (1 PLC)"=w451, "VISA resource name"=w452) -> ("error out"=w443:errorcluster, "VISA resource name out"=w441:refnum<visa-resource-name>)  [unwired: 7 in]
                          n214 = call <instrlib>:"Configure Multipoint.vi"("error in (no error)"=w443, "Trigger Count (1)"=w439, "VISA resource name"=w441) -> ("error out"=w447:errorcluster, "VISA resource name out"=w448:refnum<visa-resource-name>)  [unwired: 7 in]
                          n215 = call <instrlib>:"Configure Trigger.vi"("Trigger Source (0: Immediate)"=w440, "error in (no error)"=w447, "VISA resource name"=w448) -> ("error out"=w446:errorcluster, "VISA resource name out"=w445:refnum<visa-resource-name>)  [unwired: 7 in]
                          n216 = call <instrlib>:"Enable Output.vi"("error in (no error)"=w446, "Enable Output (T: Enable)"=TRUE, "VISA resource name"=w445) -> ("error out"=w442:errorcluster)  [unwired: 7 in, 1 out]
                        }
                      }
                    }
                    n217 = Merge Errors(w408) -> (w401:errorcluster)
                    "Path" <- w403
                  }
                  frame Error {
                  }
                }
                n218 = Strip Path(path=w371) -> (name=→"Filename":string)  [unwired: 1 out]
                n219 = case shown="No Error" w365 {
                  selector: w365 -> [w381 w394]
                  tunnel: w367 -> [_ w390]
                  tunnel: w366 -> [w385 _]
                  frame No Error {
                    n220 = local read "Number of Instruments"() -> (w379:u64)
                    n221 = call <vilib>:"Create Rendezvous.vi"("error in (no error)"=w381, "size (2)"=w379) -> ("error out"=w380:errorcluster, "rendezvous"=→"rendezvous":T1)  [unwired: 3 in, 1 out]
                    n222 = call "set control visibility.vi"("error in"=w380, "Disabled"=T4."Enabled", "Controls Reference Array"=w385) -> ("error out"=w383:errorcluster)  [unwired: 1 in]
                    n223 = call "Get date and time in seconds sequential.vi"("error in (no error)"=w383) -> ("error out"=w386:errorcluster, "current time"=w388:timestamp)  [unwired: 1 in]
                    n224 = To Double Precision Float(number=w388) -> (double precision float=→"start time":dbl)
                    n225 = property on="Running" class="Bool (strict)"(error in=w386, "Value"=TRUE) -> ()  [unwired: 1 in, 2 out]
                  }
                  frame Error {
                    n226 = call <vilib>:"General Error Handler.vi"("error in (no error)"=w394) -> ("error out"=w393:errorcluster)  [unwired: 10 in, 4 out]
                    n227 = call <vilib>:"Clear Errors.vi"("error in (no error)"=w393) -> ("error out"=w392:errorcluster)  [unwired: 5 in, 1 out]
                    n228 = call "set control visibility.vi"("error in"=w392, "Disabled"=T4."Enabled", "Controls Reference Array"=w390) -> ()  [unwired: 1 in, 1 out]
                  }
                }
              }
            }
          }
          event "Stop": Value Change {
            n229 = event-data() -> ()  [unwired: 1 in, 6 out]
            n230 = case shown="True" "Stop" {
              tunnel: w471 -> [_ w486]
              tunnel: [_ w472] -> w470
              tunnel: w467 -> [_ w479]
              frame False {
              }
              frame True {
                n231 = property on="Running" class="Bool (strict)"() -> (error out=w481:errorcluster, "Value"=w482:bool)  [unwired: 2 in, 1 out]
                n232 = case shown="True" w482 {
                  tunnel: [w487 w491] -> w483
                  tunnel: w481 -> [w487 w490]
                  frame False {
                  }
                  frame True {
                    n233 = local read "Instrument Config"() -> (w488:T2[])
                    n234 = Array Size(array=w488) -> (size(s)=w489:i32)
                    n235 = for {
                      N: w489 -> [_]
                      tunnel: w488 -> [w496] mode=indexing
                      tunnel: [w493] -> w491
                      tunnel: w490 -> [w492]
                      n236 = Unbundle By Name(w496) -> ("Instrument Address"=w494:refnum<visa-resource-name>, "Instrument Type"=w495:T6)
                      n237 = case shown="\"24XX SMU\"" w495 {
                        tunnel: w494 -> [w499 w502]
                        tunnel: [w498 w501] -> w493
                        tunnel: w492 -> [w497 w500]
                        frame "648X Picoammeter", Default {
                          n238 = call <instrlib>:"Abort.vi"("VISA resource name"=w499, "error in (no error)"=w497) -> ("error out"=w498:errorcluster)  [unwired: 12 in, 1 out]
                        }
                        frame "24XX SMU" {
                          n239 = call <instrlib>:"Abort.vi"("error in (no error)"=w500, "VISA resource name"=w502) -> ("error out"=w501:errorcluster)  [unwired: 8 in, 1 out]
                        }
                      }
                    }
                  }
                }
                n240 = call <vilib>:"Clear Errors.vi"("error in (no error)"=w483) -> ("error out"=w476:errorcluster)  [unwired: 5 in, 1 out]
                n241 = property on="Running" class="Bool (strict)"(error in=w476, "Value"=FALSE) -> (error out=w475:errorcluster)  [unwired: 1 in, 1 out]
                n242 = call "set control visibility.vi"("error in"=w475, "Disabled"=T4."Enabled", "Controls Reference Array"=w486) -> ("error out"=w477:errorcluster)  [unwired: 1 in]
                n243 = local read "rendezvous"() -> (w484:T1)
                n244 = call "set control visibility.vi"("error in"=w477, "Disabled"=T4."Disabled and Grayed Out", "Controls Reference Array"=w479) -> ("error out"=w474:errorcluster)  [unwired: 1 in]
                n245 = call <vilib>:"Destroy Rendezvous.vi"("error in (no error)"=w474, "rendezvous"=w484) -> ("error out"=w473:errorcluster)  [unwired: 4 in, 1 out]
                n246 = call <vilib>:"Clear Errors.vi"("error in (no error)"=w473) -> ("error out"=w472:errorcluster)  [unwired: 5 in, 1 out]
              }
            }
            n247 = property on="Stop" class="Bool (strict)"(error in=w470, "Value"=FALSE) -> ()  [unwired: 1 in, 2 out]
          }
          event "Exit": Value Change {
            w505 = T3 {"Number of Instruments"=0, "Instrument Config"=[], "Integration Speed"=0, "Measurement Mode"=0, "Number of Trials\nMax 2500 for remote"=0, "Trigger type"=enum."Software", "Trigger Hardware Address"=""}  # Save cluster
            n248 = event-data() -> ()  [unwired: 1 in, 6 out]
            n249 = local read "Number of Trials\nMax 2500 for remote"() -> (w508:i16)
            n250 = local read "Trigger Hardware Address"() -> (w503:refnum<visa-resource-name>)
            n251 = local read "Number of Instruments"() -> (w512:u64)
            n252 = local read "Instrument Config"() -> (w511:T2[])
            n253 = local read "Integration Speed"() -> (w510:u16)
            n254 = local read "Looping Mode"() -> (w509:enum16{"Remote looping", "Local looping"})
            n255 = local read "Trigger type"() -> (w504:enum16{"Software", "Hardware"})
            n256 = Bundle By Name(cluster=w505, "Number of Instruments"=w512, "Instrument Config"=w511, "Integration Speed"=w510, "Measurement Mode"=w509, "Number of Trials\nMax 2500 for remote"=w508, "Trigger type"=w504, "Trigger Hardware Address"=w503) -> (w507:T3)
          }
        }
      }
      n257 = Flatten To XML(6:w58) -> (2:w57:string)
      n258 = call-poly <vilib>:"Write to XML File.vi"("error in (no error)"=w56, "XML Input"=w57, "XML File Path"=w55) -> ()  [unwired: 6 in, 3 out]
    }
    frame Error {
      n259 = call <vilib>:"General Error Handler.vi"("error in (no error)"=w514) -> ()  [unwired: 10 in, 5 out]
    }
  }
